vi "RIGOL DS1000 Series Acquire Continuous Waveform.vi"() -> ()   [LabVIEW 2018]
doc: "This example shows how to use autosetup and acquire a waveform on a single channel."
uses:
  <instrlib>/RIGOL DS1000 Series/Public/Data/Read (Single Waveform).vi
  <instrlib>/RIGOL DS1000 Series/RIGOL DS1000 Series.lvlib
panel:
  in  "Channel (0: Channel 1)":u16(ring) items=["Channel 1", "Channel 2", "Channel 3", "Channel 4"]
  in  "Stop":bool
  in  "Timeout (10000 ms)":u32=10000
  out "Waveform Data":waveform(dbl)(graph)
  in  "VISA resource name":refnum<visa-resource-name>
  # "(c) 2010-2012, RIGOL Technologies, Inc.  All Rights Reserved."
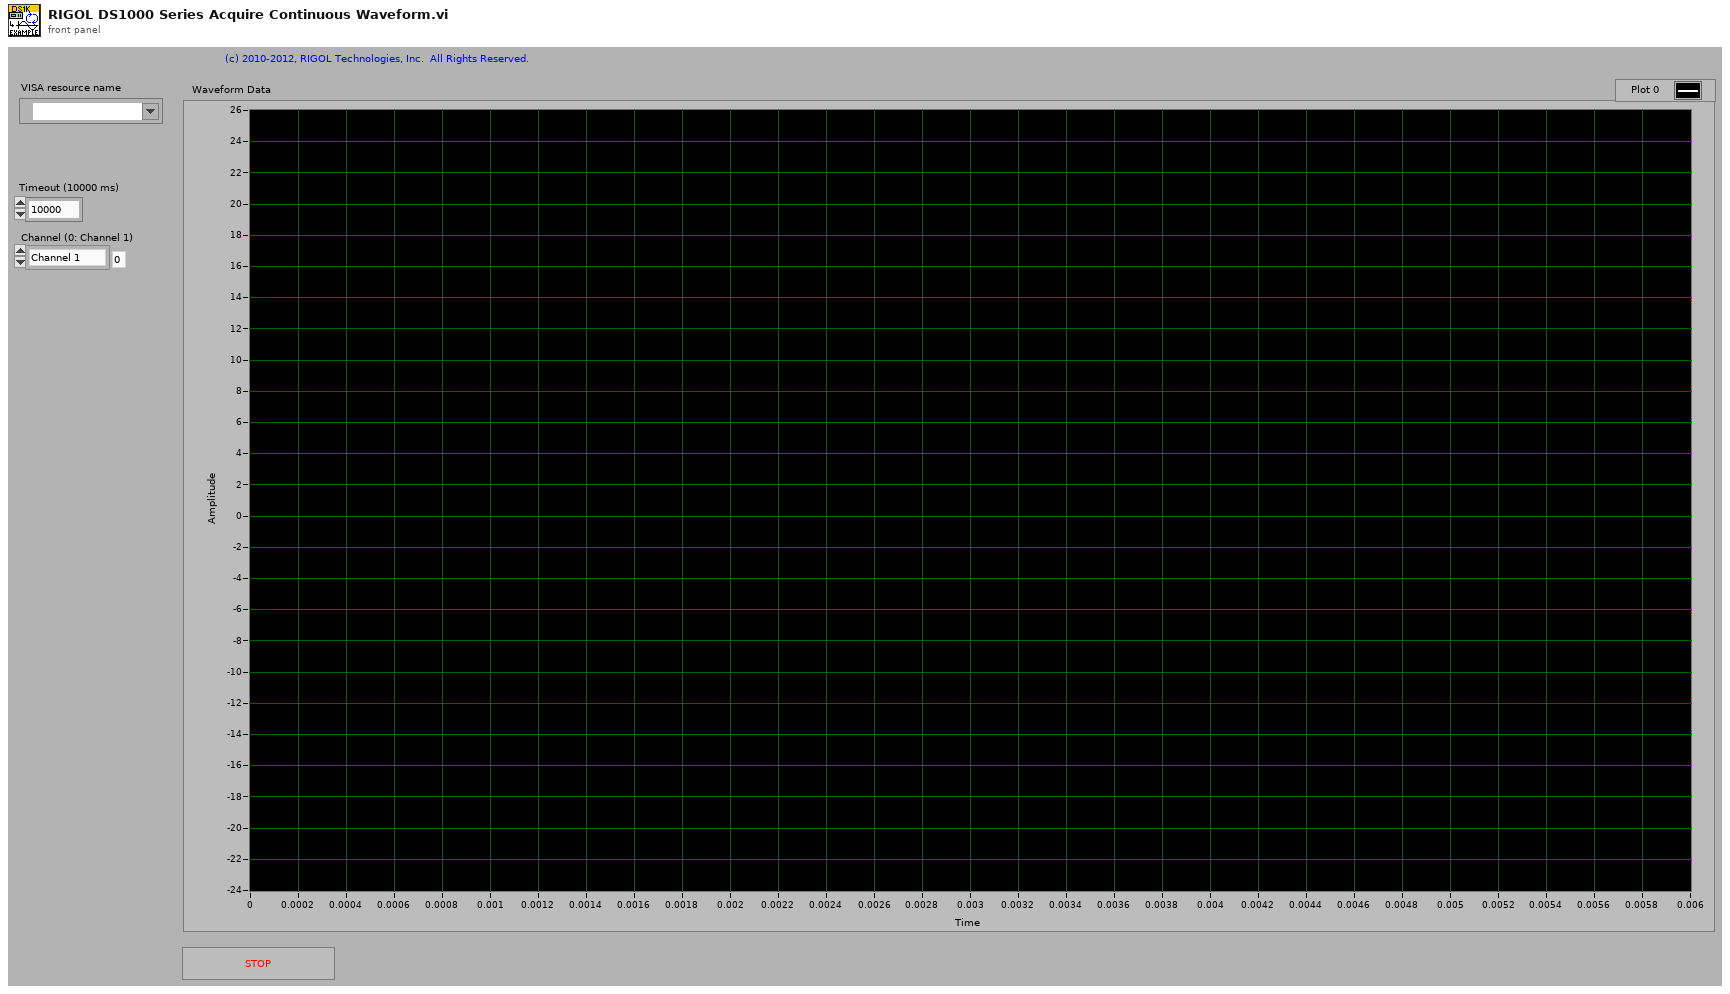
[diagram p1: front panel]
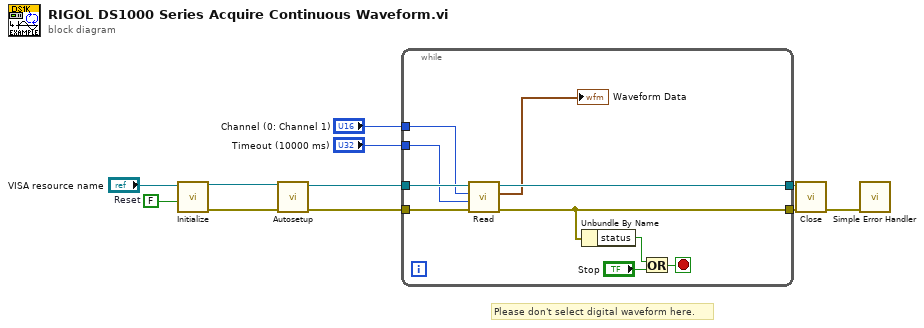
[diagram p0: block diagram]
diagram:
  w1 = FALSE  # Reset
  # "Please don't select digital waveform here."
  n1 = call <instrlib>:"Initialize.vi"("Reset (True)"=w1, "VISA resource name"="VISA resource name") -> ("error out"=w6:errorcluster, "VISA resource name out"=w5:refnum<visa-resource-name>)  [unwired: 2 in, 6 out]
  n2 = call <instrlib>:"Autosetup.vi"("error in (no error)"=w6, "VISA resource name"=w5) -> ("error out"=w3:errorcluster, "VISA resource name out"=w4:refnum<visa-resource-name>)  [unwired: 8 out]
  n3 = while {
    tunnel: w4 -> [w21]
    tunnel: w3 -> [w20]
    tunnel: [w19] -> w10
    tunnel: [w17] -> w9
    tunnel: "Timeout (10000 ms)" -> [w13]
    tunnel: "Channel (0: Channel 1)" -> [w14]
    stop <- w18 stop-if-true
    n4 = call-poly <instrlib>:"Read.vi"("error in (no error)"=w20, "Timeout (10000 ms)"=w13, "Channel (0: Channel 1)"=w14, "VISA resource name"=w21) -> ("error out"=w17:errorcluster, "Waveform Data"=→"Waveform Data":waveform(dbl), "VISA resource name out"=w19:refnum<visa-resource-name>)  [unwired: 5 out]
    n5 = Unbundle By Name(w17) -> ("status"=w16:bool)
    n6 = Or(x=w16, y="Stop") -> (x .or. y?=w18:bool)
  }
  n7 = call <instrlib>:"Close.vi"("error in (no error)"=w9, "VISA resource name"=w10) -> ("error out"=w11:errorcluster)  [unwired: 9 out]
  n8 = call <vilib>:"Simple Error Handler.vi"("error in (no error)"=w11) -> ()  [unwired: 1 in, 8 out]
